vi "set_state.vi"(8 "error in (no error)":errorcluster, 10 "state":bool, 11 "GenericDigitalOut in":refnum<class "GenericDigitalOut.lvclass">) -> (0 "error out":errorcluster, 3 "GenericDigitalOut out":refnum<class "GenericDigitalOut.lvclass">)   [LabVIEW 2010, in "GenericDigitalOut.lvclass"]
uses:
  GenericDigitalOut.lvclass
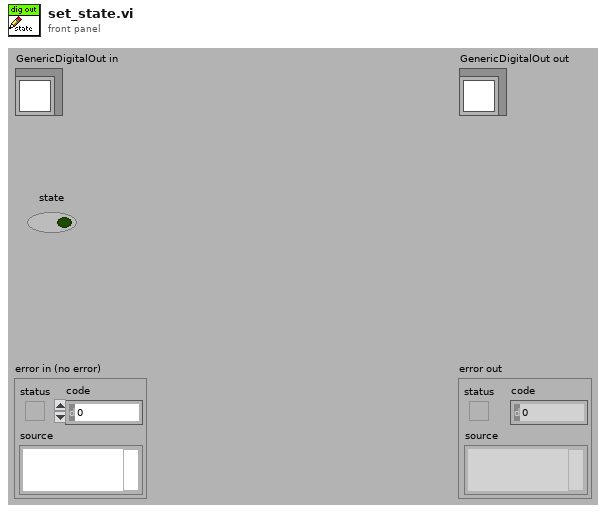
[diagram p1: front panel]
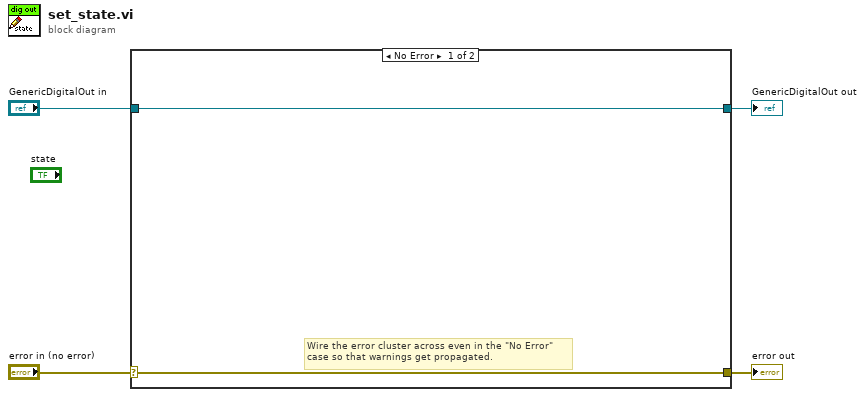
[diagram p0: block diagram]
diagram:
  n1 = case shown="No Error" "error in (no error)" {
    selector: "error in (no error)" -> [w5 w8]
    tunnel: [w5 w8] -> w3
    tunnel: [w6 w7] -> w1
    tunnel: "GenericDigitalOut in" -> [w6 w7]
    frame No Error {
      # "Wire the error cluster across even in the \"No Error\"\ncase so that warnings get propagated."
    }
    frame Error {
    }
  }
  "error out" <- w3
  "GenericDigitalOut out" <- w1
